vi "Field Retrieve Record.vi"(8 "error in (no error)":errorcluster, 11 "Statement Refnum":T1) -> (0 "error out":errorcluster, 2 "Field Record":T2={"ixField"=0, "iSequenceOrder"=0, "sxFieldId"="", "sxSequenceId"="", "sDisplayName"="", "sValue"="", "sUnits"="", "nDataType"=enum."timestamp", "nNextItem"=enum."Reset", "fSystem"=FALSE, "fSystemValue"=FALSE, "fRequired"=FALSE, "fSetAtTest"=FALSE, "fTestField"=FALSE, "fDeleted"=FALSE, "fIndexed"=FALSE, "fFreeList"=FALSE}, 3 "Statement Refnum":T1)   [LabVIEW 2011]
uses:
  Field Record.ctl
  Field DataTypes.ctl
  Field NextItem.ctl
  Summitek EXT/ODBC/SQL Controls/Statement Refnum.ctl
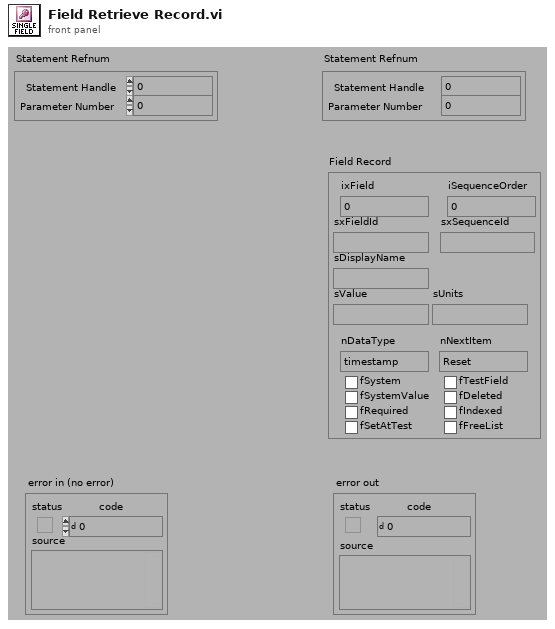
[diagram p1: front panel]
types:
  T1 = typedef "Statement Refnum.ctl" = cluster{"Statement Handle":i32, "Parameter Number":u16}
  T2 = typedef "Field Record.ctl" = cluster{"ixField":i32, "iSequenceOrder":i32, "sxFieldId":string, "sxSequenceId":string, "sDisplayName":string, "sValue":string, "sUnits":string, "nDataType":T3, "nNextItem":T4, "fSystem":bool, "fSystemValue":bool, "fRequired":bool, "fSetAtTest":bool, "fTestField":bool, "fDeleted":bool, "fIndexed":bool, "fFreeList":bool}
  T3 = typedef "Field DataTypes.ctl" = enum32{"text", "numeric", "list", "timestamp", "boolean"}
  T4 = typedef "Field NextItem.ctl" = enum32{"Reset", "Retain", "Auto-Increment"}
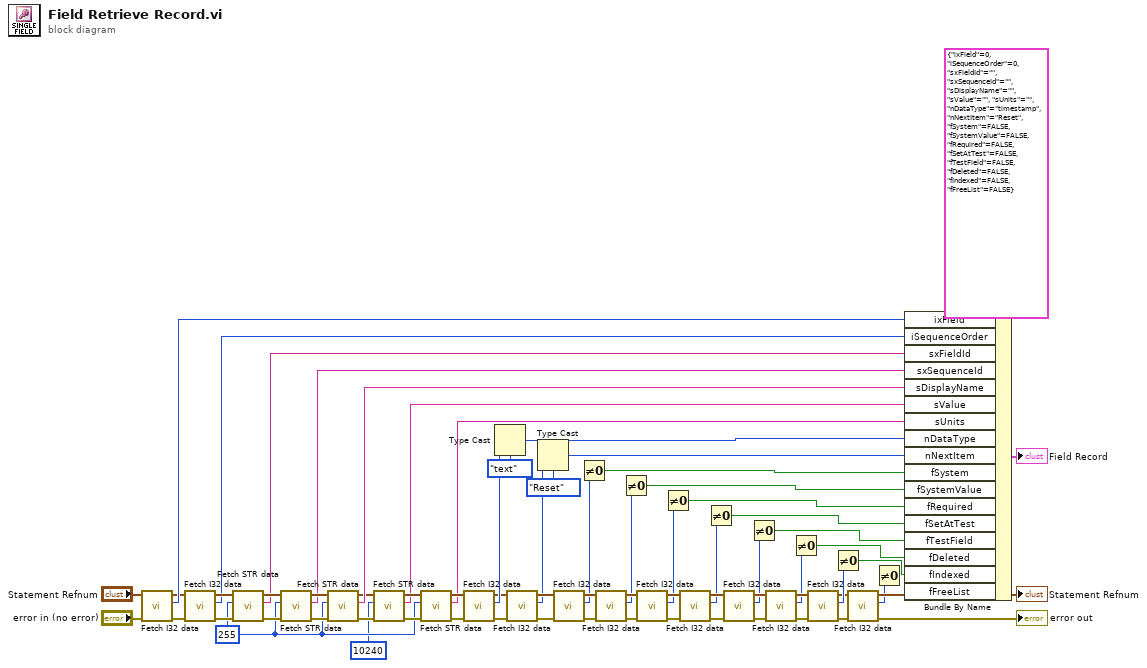
[diagram p0: block diagram]
diagram:
  w46 = 255 ("Buffer Size")
  n1 = call "Fetch I32 data.vi"("error in (no error)"="error in (no error)", "Statement Refnum"="Statement Refnum") -> ("error out"=w58:errorcluster, "Data"=w60:i32, "Statement Refnum"=w56:T1)  [unwired: 3 out]
  n2 = call "Fetch I32 data.vi"("error in (no error)"=w58, "Statement Refnum"=w56) -> ("error out"=w57:errorcluster, "Data"=w54:i32, "Statement Refnum"=w55:T1)  [unwired: 3 out]
  n3 = call "Fetch STR data.vi"("error in (no error)"=w57, "Buffer Size"=w46, "Statement Refnum"=w55) -> ("error out"=w62:errorcluster, "Data"=w53:string, "Statement Refnum"=w61:T1)  [unwired: 2 out]
  n4 = call "Fetch STR data.vi"("error in (no error)"=w62, "Buffer Size"=w46, "Statement Refnum"=w61) -> ("error out"=w69:errorcluster, "Data"=w52:string, "Statement Refnum"=w68:T1)  [unwired: 2 out]
  n5 = call "Fetch STR data.vi"("error in (no error)"=w69, "Buffer Size"=w46, "Statement Refnum"=w68) -> ("error out"=w49:errorcluster, "Data"=w51:string, "Statement Refnum"=w50:T1)  [unwired: 2 out]
  n6 = call "Fetch STR data.vi"("error in (no error)"=w49, "Buffer Size"=10240, "Statement Refnum"=w50) -> ("error out"=w48:errorcluster, "Data"=w45:string, "Statement Refnum"=w47:T1)  [unwired: 2 out]
  n7 = call "Fetch STR data.vi"("error in (no error)"=w48, "Buffer Size"=w46, "Statement Refnum"=w47) -> ("error out"=w64:errorcluster, "Data"=w44:string, "Statement Refnum"=w65:T1)  [unwired: 2 out]
  n8 = call "Fetch I32 data.vi"("error in (no error)"=w64, "Statement Refnum"=w65) -> ("error out"=w12:errorcluster, "Data"=w42:i32, "Statement Refnum"=w14:T1)  [unwired: 3 out]
  n9 = Type Cast(type=Field_DataTypes."text" ("nDataType"), x=w42) -> (*(type *) &x=w41:T3)
  n10 = call "Fetch I32 data.vi"("error in (no error)"=w12, "Statement Refnum"=w14) -> ("error out"=w11:errorcluster, "Data"=w10:i32, "Statement Refnum"=w13:T1)  [unwired: 3 out]
  n11 = Type Cast(type=Field_NextItem."Reset" ("nNextItem"), x=w10) -> (*(type *) &x=w15:T4)
  n12 = call "Fetch I32 data.vi"("error in (no error)"=w11, "Statement Refnum"=w13) -> ("error out"=w28:errorcluster, "Data"=w17:i32, "Statement Refnum"=w29:T1)  [unwired: 3 out]
  n13 = Not Equal To 0?(x=w17) -> (x != 0?=w16:bool)
  n14 = call "Fetch I32 data.vi"("error in (no error)"=w28, "Statement Refnum"=w29) -> ("error out"=w39:errorcluster, "Data"=w27:i32, "Statement Refnum"=w34:T1)  [unwired: 3 out]
  n15 = Not Equal To 0?(x=w27) -> (x != 0?=w26:bool)
  n16 = call "Fetch I32 data.vi"("error in (no error)"=w39, "Statement Refnum"=w34) -> ("error out"=w36:errorcluster, "Data"=w21:i32, "Statement Refnum"=w33:T1)  [unwired: 3 out]
  n17 = Not Equal To 0?(x=w21) -> (x != 0?=w25:bool)
  n18 = call "Fetch I32 data.vi"("error in (no error)"=w36, "Statement Refnum"=w33) -> ("error out"=w38:errorcluster, "Data"=w20:i32, "Statement Refnum"=w32:T1)  [unwired: 3 out]
  n19 = Not Equal To 0?(x=w20) -> (x != 0?=w24:bool)
  n20 = call "Fetch I32 data.vi"("error in (no error)"=w38, "Statement Refnum"=w32) -> ("error out"=w35:errorcluster, "Data"=w19:i32, "Statement Refnum"=w31:T1)  [unwired: 3 out]
  n21 = Not Equal To 0?(x=w19) -> (x != 0?=w23:bool)
  n22 = call "Fetch I32 data.vi"("error in (no error)"=w35, "Statement Refnum"=w31) -> ("error out"=w37:errorcluster, "Data"=w18:i32, "Statement Refnum"=w30:T1)  [unwired: 3 out]
  n23 = Not Equal To 0?(x=w18) -> (x != 0?=w22:bool)
  n24 = call "Fetch I32 data.vi"("error in (no error)"=w37, "Statement Refnum"=w30) -> ("error out"=w5:errorcluster, "Data"=w9:i32, "Statement Refnum"=w7:T1)  [unwired: 3 out]
  n25 = Not Equal To 0?(x=w9) -> (x != 0?=w8:bool)
  n26 = call "Fetch I32 data.vi"("error in (no error)"=w5, "Statement Refnum"=w7) -> ("error out"=→"error out":errorcluster, "Data"=w3:i32, "Statement Refnum"=→"Statement Refnum":T1)  [unwired: 3 out]
  n27 = Not Equal To 0?(x=w3) -> (x != 0?=w2:bool)
  n28 = Bundle By Name(cluster=T2 {"ixField"=0, "iSequenceOrder"=0, "sxFieldId"="", "sxSequenceId"="", "sDisplayName"="", "sValue"="", "sUnits"="", "nDataType"=enum."timestamp", "nNextItem"=enum."Reset", "fSystem"=FALSE, "fSystemValue"=FALSE, "fRequired"=FALSE, "fSetAtTest"=FALSE, "fTestField"=FALSE, "fDeleted"=FALSE, "fIndexed"=FALSE, "fFreeList"=FALSE} ("Field Data Information"), "ixField"=w60, "iSequenceOrder"=w54, "sxFieldId"=w53, "sxSequenceId"=w52, "sDisplayName"=w51, "sValue"=w45, "sUnits"=w44, "nDataType"=w41, "nNextItem"=w15, "fSystem"=w16, "fSystemValue"=w26, "fRequired"=w25, "fSetAtTest"=w24, "fTestField"=w23, "fDeleted"=w22, "fIndexed"=w8, "fFreeList"=w2) -> (→"Field Record":T2)
